vi "Packetize.vi"(8 "Error In":errorcluster, 9 "ARGS":u8[](array[numeric]), 10 "CMD":u16, 11 "LINX Device Config":T1) -> (0 "Error Out":errorcluster, 2 "Packet":string, 3 "LINX Decice Config":T1)   [LabVIEW 2011, in "LVH-LINX.lvlib"]
doc: "This VI takes a LINX command and arguments and builds a LINX packet."
uses:
  LVH-LINX.lvlib
  Type Defs/LINX Device Config.ctl
  Type Defs/Interface.ctl
  Type Defs/TCP Config.ctl
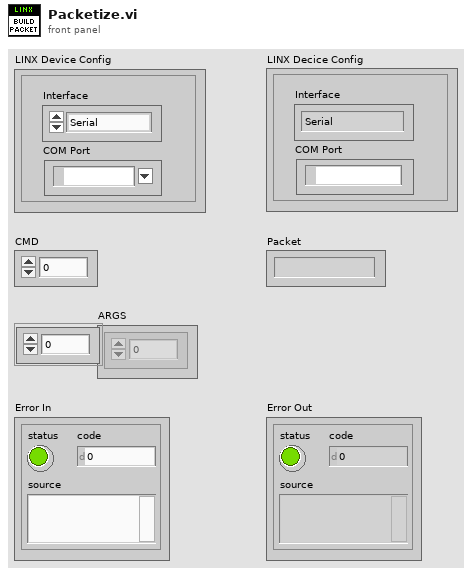
[diagram p1: front panel]
types:
  T1 = typedef "LVH-LINX.lvlib/LINX Device Config.ctl" = cluster{"Interface":T2, "COM Port":refnum<visa-resource-name>, "Packet Number":u16, "TCP Configuration":T3}
  T2 = typedef "LVH-LINX.lvlib/Interface.ctl" = enum16{"Serial", "TCP"}
  T3 = typedef "LVH-LINX.lvlib/TCP Config.ctl" = cluster{"IP Address":string, "Port":dbl}
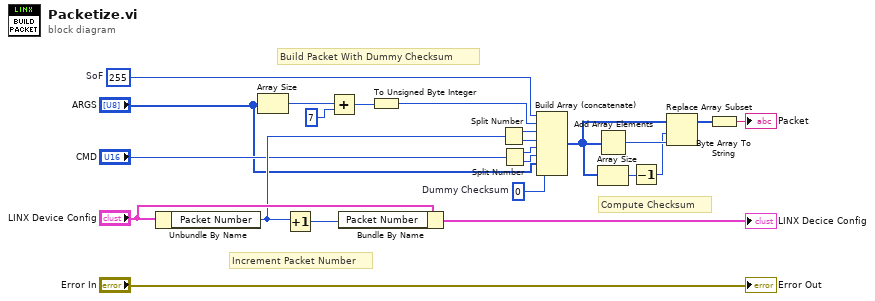
[diagram p0: block diagram]
diagram:
  w9 = u8 0  # Dummy Checksum
  w19 = u8 255  # SoF
  # "Increment Packet Number"
  # "Build Packet With Dummy Checksum"
  # "Compute Checksum"
  n1 = Unbundle By Name("LINX Device Config") -> ("Packet Number"=w16:u16)
  n2 = Array Size(array="ARGS") -> (size(s)=w21:i32)
  n3 = Increment(x=w16) -> (x+1=w22:u16)
  n4 = Add(x=w21, y=7) -> (x+y=w18:i32)
  n5 = Bundle By Name(cluster="LINX Device Config", "Packet Number"=w22) -> (→"LINX Decice Config":T1)
  n6 = To Unsigned Byte Integer(number=w18) -> (unsigned 8bit integer=w17:u8)
  n7 = Split Number(x=w16) -> (hi(x)=w15:u8, lo(x)=w14:u8)
  n8 = Split Number(x="CMD") -> (hi(x)=w13:u8, lo(x)=w12:u8)
  n9 = Build Array (concatenate)(w19, w17, w15, w14, w13, w12, "ARGS", w9) -> (w8:u8[])
  n10 = Add Array Elements(numeric array=w8) -> (sum=w7:u8)
  n11 = Array Size(array=w8) -> (size(s)=w2:i32)
  n12 = Decrement(x=w2) -> (x-1=w1:i32)
  n13 = Replace Array Subset(array=w8, new element=w7, index=w1) -> (w4:u8[])
  n14 = Byte Array To String(unsigned byte array=w4) -> (string=→"Packet":string)
  "Error Out" <- "Error In"
